vi "KE622x -- Set Results Format tmp.vi"(0 "Resource In":refnum<visa-resource-name>, 1 "Check For SCPI Errors? (T)":bool=TRUE, 7 "Results Format":T1={"Results Format"=enum."ASCII", "Bin Byte Order"=enum."Swapped"}, 11 "error in (no error)":errorcluster) -> (4 "Resource Out (dupl)":refnum<visa-resource-name>, 15 "error out":errorcluster)   [LabVIEW 2014, in "Keithley 622x tmp.lvlib"]
doc: "Sets the bus transfer format for measurements sent from the instrument to the PC, either ASCII, Single Precision, or Double Precision. In addition, it is also possible to change the byte order in either Single or Double Precision formats. For maximum bus transfer speeds, use Single Precision."
uses:
  Keithley 622x tmp.lvlib
  Typedefs/KE622x -- Results Format.ctl
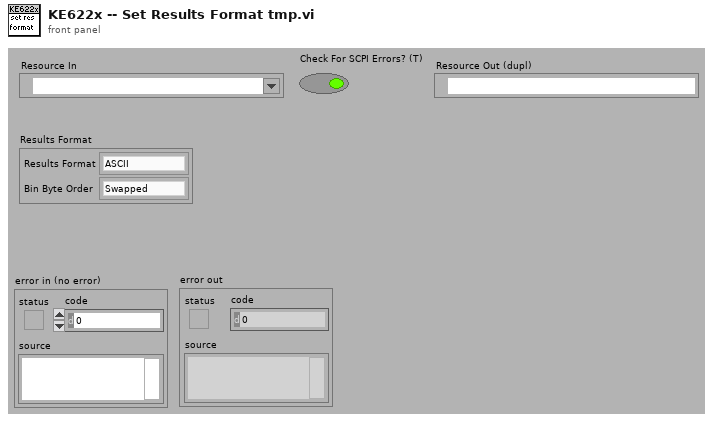
[diagram p1: front panel]
types:
  T1 = typedef "Keithley 622x tmp.lvlib/KE622x -- Results Format.ctl" = cluster{"Results Format":enum16{"ASCII", "Single Prec Bin", "Double Prec Bin"}, "Bin Byte Order":enum16{"Normal", "Swapped"}}
  T2 = enum16{"ASCII", "Single Prec Bin", "Double Prec Bin"}
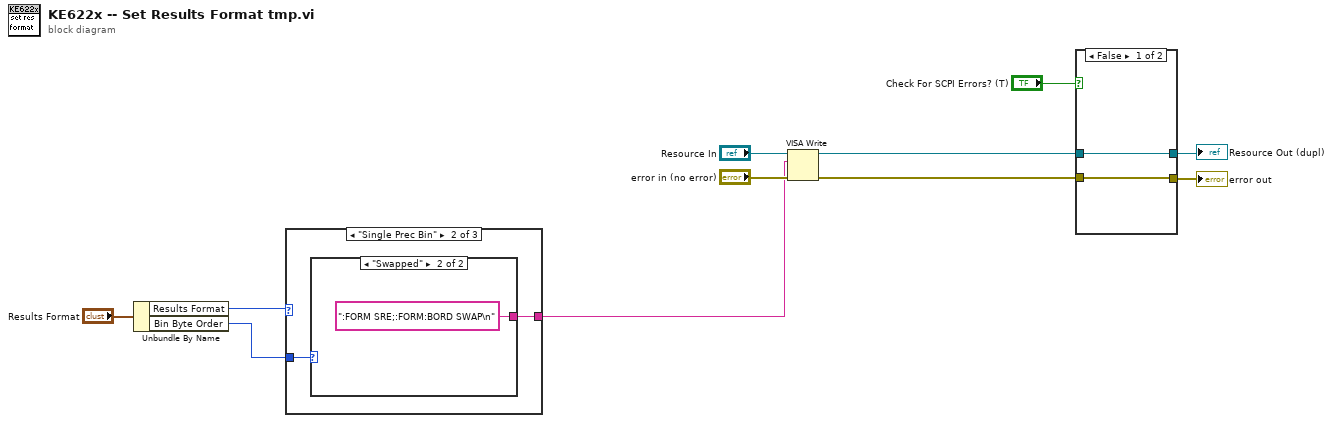
[diagram p0: block diagram]
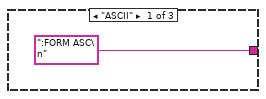
[diagram p2: hidden frame]
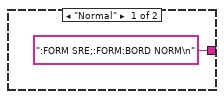
[diagram p3: hidden frame]
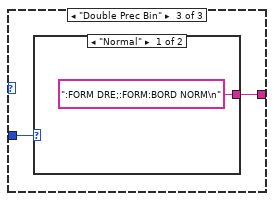
[diagram p4: hidden frame]
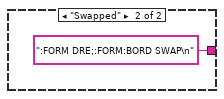
[diagram p5: hidden frame]
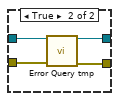
[diagram p6: hidden frame]
diagram:
  n1 = Unbundle By Name("Results Format") -> ("Results Format"=w3:T2, "Bin Byte Order"=w2:enum16{"Normal", "Swapped"})
  n2 = case shown="\"Single Prec Bin\"" w3 {
    tunnel: [":FORM ASC\n" w13 w17] -> w1
    tunnel: w2 -> [_ w14 w18]
    frame "ASCII" {
    }
    frame "Single Prec Bin" {
      n3 = case shown="\"Swapped\"" w14 {
        tunnel: [":FORM SRE;:FORM:BORD NORM\n" ":FORM SRE;:FORM:BORD SWAP\n"] -> w13
        frame "Normal" {
        }
        frame "Swapped" {
        }
      }
    }
    frame "Double Prec Bin" {
      n4 = case shown="\"Normal\"" w18 {
        tunnel: [":FORM DRE;:FORM:BORD NORM\n" ":FORM DRE;:FORM:BORD SWAP\n"] -> w17
        frame "Normal" {
        }
        frame "Swapped" {
        }
      }
    }
  }
  n5 = VISA Write(VISA resource name="Resource In", write buffer=w1, error in (no error)="error in (no error)") -> (VISA resource name out=w8:refnum<visa-resource-name>, error out=w7:errorcluster)  [unwired: 1 out]
  n6 = case shown="False" "Check For SCPI Errors? (T)" {
    tunnel: w8 -> [w22 w26]
    tunnel: w7 -> [w21 w25]
    tunnel: [w21 w24] -> w5
    tunnel: [w22 w23] -> w6
    frame False {
    }
    frame True {
      n7 = call "Error Query tmp.vi"("VISA Resource In"=w26, "error in (no error)"=w25) -> ("VISA Resource Out (dupl)"=w23:refnum<visa-resource-name>, "error out"=w24:errorcluster)  [unwired: 10 in, 2 out]
    }
  }
  "Resource Out (dupl)" <- w6
  "error out" <- w5
